vi "Post-Smite Hook.vi"(8 "Error In":errorcluster) -> (0 "Error Out":errorcluster)   [LabVIEW 2018, in "Tests.lvlib" / "Toolkit.lvlib" / "Integration.lvlib"]
uses:
  Integration.lvlib
  Support/Smite Target.vi
  Hooks/Post-Smite.vi
  <vilib>/addons/_JKI Toolkits/Caraya/classes/Test/Test.lvclass
  Tests.lvlib
  <vilib>/addons/_JKI Toolkits/Caraya/classes/Assert/Assert.lvclass
  src/Toolkit/Toolkit.lvlib
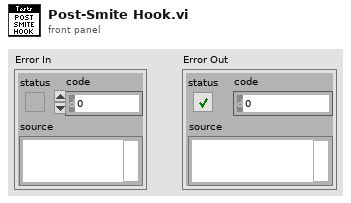
[diagram p1: front panel]
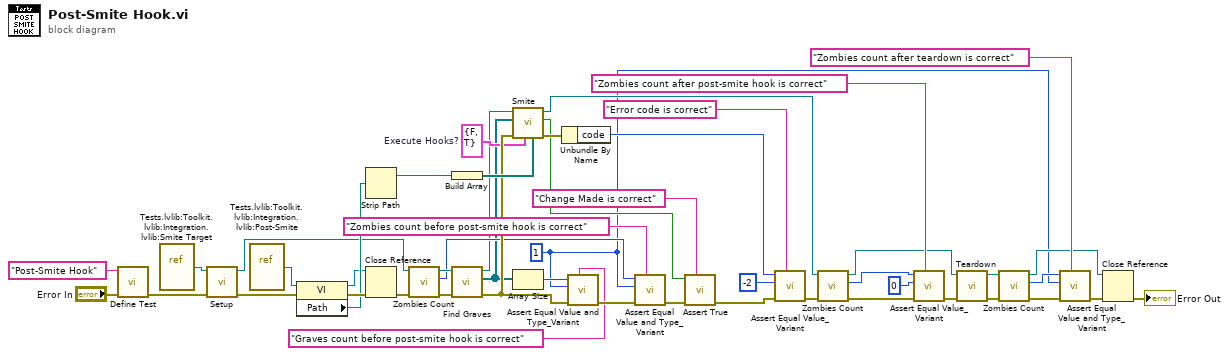
[diagram p0: block diagram]
diagram:
  w2 = 1 ("size(s)")
  w19 = cluster{"Pre":bool, "Post":bool} {"Pre"=FALSE, "Post"=TRUE}  # Execute Hooks?
  n1 = call <vilib>:"Define Test.vi"("error in (no error)"="Error In", "Label (VI Title)"="Post-Smite Hook") -> ("error out"=w44:errorcluster)  [unwired: 9 in]
  n2 = vi-ref "Tests.lvlib:Toolkit.lvlib:Integration.lvlib:Smite Target.vi"() -> (w8:refnum<vi>)
  n3 = call "Setup.vi"("Error In"=w44, "VI In"=w8) -> ("Error Out"=w36:errorcluster, "VI Out"=w28:refnum<vi>)  [unwired: 8 in]
  n4 = vi-ref "Tests.lvlib:Toolkit.lvlib:Integration.lvlib:Post-Smite.vi"() -> (w7:refnum<vi>)
  n5 = property class="VI"(reference=w7, error in=w36) -> (reference out=w32:refnum<vi>, error out=w35:errorcluster, "Path"=w34:path)
  n6 = Strip Path(path=w34) -> (stripped path=w33:path)  [unwired: 1 out]
  n7 = Close Reference(reference=w32, error in (no error)=w35) -> (error out=w15:errorcluster)
  n8 = call "Zombies Count.vi"("Error In"=w15, "Test Target In"=w28) -> ("Error Out"=w14:errorcluster, "Zombies Count"=w9:i32, "Test Target Out"=w16:refnum<vi>)  [unwired: 7 in]
  n9 = Build Array(w33) -> (w29:path[])
  n10 = call "Find Graves.vi"("Error In"=w14, "VI In"=w16) -> ("Error Out"=w27:errorcluster, "Graves"=w5:refnum<vi>[], "VI Out"=w6:refnum<vi>)  [unwired: 7 in]
  n11 = call "Smite.vi"("Hook Search Path"=w29, "Execute Hooks?"=w19, "Error In"=w27, "Graves"=w5, "VI In"=w6) -> ("Error Out"=w25:errorcluster, "Change Made?"=w3:bool, "VI Out"=w4:refnum<vi>)  [unwired: 4 in]
  n12 = Array Size(array=w5) -> (size(s)=w26:i32)
  n13 = Unbundle By Name(w25) -> ("code"=w31:i32)
  n14 = call <vilib>:"Assert Equal Value and Type_Variant.vi"("Label"="Graves count before post-smite hook is correct", "error in (no error)"=w27, "Y"=w2, "X"=w26) -> ("error out"=w13:errorcluster)  [unwired: 7 in]
  n15 = call <vilib>:"Assert Equal Value and Type_Variant.vi"("Label"="Zombies count before post-smite hook is correct", "error in (no error)"=w13, "Y"=w2, "X"=w9) -> ("error out"=w12:errorcluster)  [unwired: 7 in]
  n16 = call <vilib>:"Assert True.vi"("Label"="Change Made is correct", "error in (no error)"=w12, "True?"=w3) -> ("error out"=w18:errorcluster)  [unwired: 8 in]
  n17 = call <vilib>:"Assert Equal Value_Variant.vi"("Label"="Error code is correct", "error in (no error)"=w18, "Y"=-2 ("code"), "X"=w31) -> ("error out"=w24:errorcluster)  [unwired: 7 in]
  n18 = call "Zombies Count.vi"("Error In"=w24, "Test Target In"=w4) -> ("Error Out"=w23:errorcluster, "Zombies Count"=w22:i32, "Test Target Out"=w21:refnum<vi>)  [unwired: 7 in]
  n19 = call <vilib>:"Assert Equal Value_Variant.vi"("Label"="Zombies count after post-smite hook is correct", "error in (no error)"=w23, "Y"=0 ("Zombies Count"), "X"=w22) -> ("error out"=w20:errorcluster)  [unwired: 7 in]
  n20 = call "Teardown.vi"("Error In"=w20, "VI In"=w21) -> ("Error Out"=w39:errorcluster, "VI Out"=w41:refnum<vi>)  [unwired: 8 in]
  n21 = call "Zombies Count.vi"("Error In"=w39, "Test Target In"=w41) -> ("Error Out"=w38:errorcluster, "Zombies Count"=w37:i32, "Test Target Out"=w40:refnum<vi>)  [unwired: 7 in]
  n22 = call <vilib>:"Assert Equal Value and Type_Variant.vi"("Label"="Zombies count after teardown is correct", "error in (no error)"=w38, "Y"=w2, "X"=w37) -> ("error out"=w43:errorcluster)  [unwired: 7 in]
  n23 = Close Reference(reference=w40, error in (no error)=w43) -> (error out=→"Error Out":errorcluster)
